vi "Decorate Core Actor.vi"(4 "Stop When Parent Stopped":bool=TRUE, 10 "Actor To Decorate Core Actor":refnum<class "Actor.lvclass">) -> (2 "Decorated Core Actor":refnum<class "Actor.lvclass">)   [LabVIEW 2025, in "jettl.lvlib"]
uses:
  Actor/Actor/Actor.lvclass
  Actor/Core Actor/Core Actor.lvclass
  jettl.lvlib
  Actor/Actor.lvlib
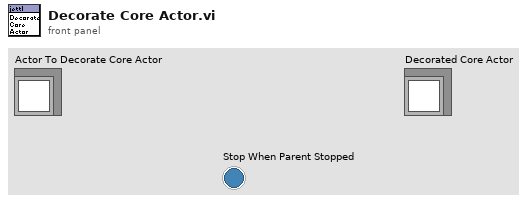
[diagram p1: front panel]
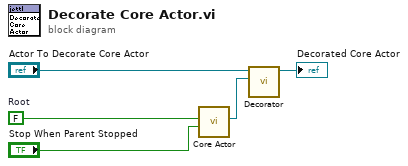
[diagram p0: block diagram]
diagram:
  w3 = FALSE  # Root
  n1 = call "Core Actor.vi"("Stop When Parent Stopped"="Stop When Parent Stopped", "Root"=w3) -> ("Actor"=w1:refnum<class "Actor.lvclass">)  [unwired: 9 in]
  n2 = call-dynamic "Decorator.vi"("Actor"=w1, "Actor in"="Actor To Decorate Core Actor") -> ("Actor out"=→"Decorated Core Actor":refnum<class "Actor.lvclass">)  [unwired: 9 in]
